vi "ResistorCalc.vi"() -> ()   [LabVIEW 2021]
panel:
  in  "2nd Band":T1(ring)
  in  "Ring":ext(ring) items=["Black", "Brown", "Red", "Orange", "Yellow", "Green", "Blue", "Violet", "Grey", "White", "Gold", "Silver"]
  out "Resistor Value":dbl
  in  "1st Band":T1(ring)
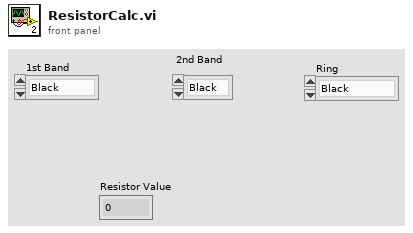
[diagram p1: front panel]
types:
  T1 = enum16{"Black", "Brown", "Red", "Orange", "Yellow", "Green", "Blue", "Violet", "Grey", "White"}
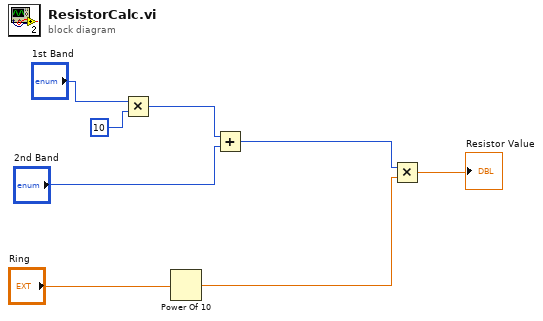
[diagram p0: block diagram]
diagram:
  n1 = Multiply(x="1st Band", y=10) -> (x*y=w7:i32)
  n2 = Power Of 10(x="Ring") -> (10^x=w4:ext)
  n3 = Add(x=w7, y="2nd Band") -> (x+y=w6:i32)
  n4 = Multiply(x=w6, y=w4) -> (x*y=→"Resistor Value":ext)
